vi "Info.vi"(8 "error in":errorcluster, 11 "Driver path":path) -> (0 "error out":errorcluster, 3 "Info":string)   [LabVIEW 2020, in "r307-python-labview-driver.lvlib"]
uses:
  r307-python-labview-driver.lvlib
panel:
  out "command line":string="cmc /c python \"%s\" ENROLL"
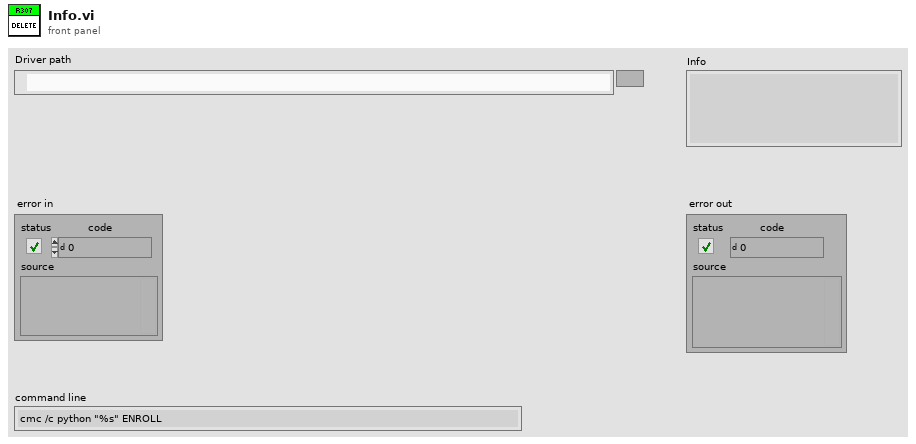
[diagram p1: front panel]
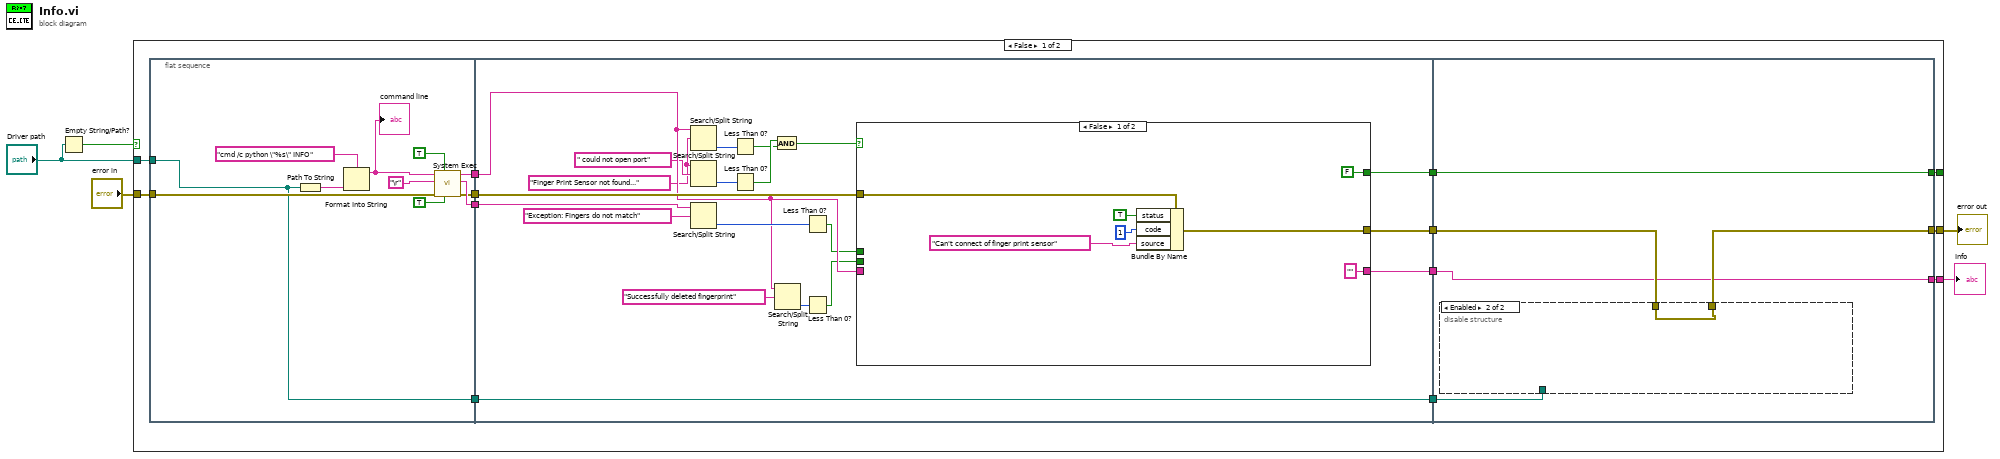
[diagram p0: block diagram]
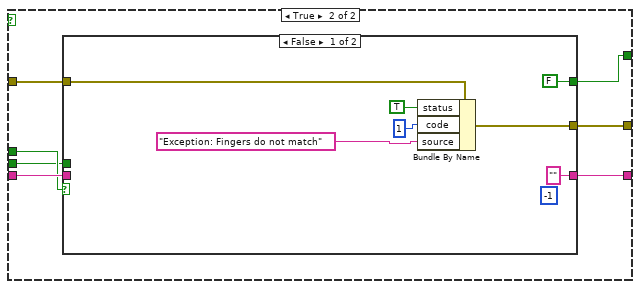
[diagram p2: hidden frame]
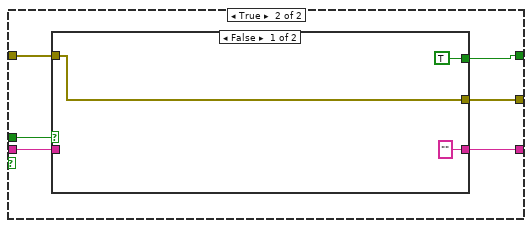
[diagram p3: hidden frame]
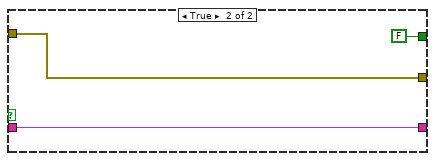
[diagram p4: hidden frame]
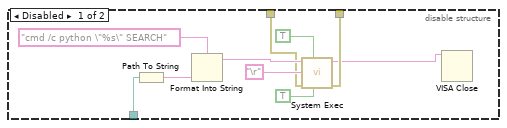
[diagram p5: hidden frame]
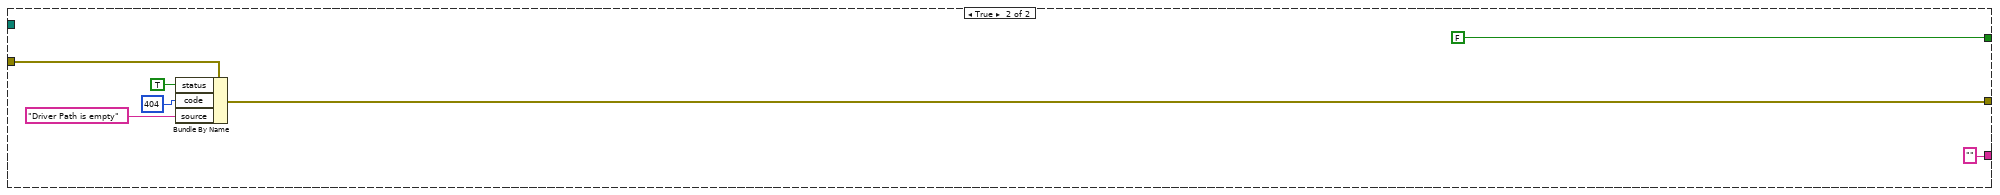
[diagram p6: hidden frame]
diagram:
  n1 = Empty String/Path?(string/path="Driver path") -> (empty?=w3:bool)
  n2 = case shown="False" w3 {
    tunnel: "Driver path" -> [w15 _]
    tunnel: "error in" -> [w14 w105]
    tunnel: [w13 w101] -> w4
    tunnel: [w12 FALSE ("Found")] -> _
    tunnel: [w7 "" ("standard output")] -> w1
    frame False {
      n3 = flat-sequence {
        tunnel: w15 -> [w19]
        tunnel: w14 -> [w21]
        tunnel: [w24] -> w18
        tunnel: [w20] -> w17
        tunnel: [w23] -> w16
        tunnel: [w19] -> w8
        tunnel: w18 -> [w48]
        tunnel: w17 -> [w47]
        tunnel: w16 -> [w41]
        tunnel: [w43] -> w11
        tunnel: [w39] -> w10
        tunnel: [w32] -> w9
        tunnel: w8 -> [w32]
        tunnel: [w30] -> w6
        tunnel: [w87] -> w12
        tunnel: [w84] -> w13
        tunnel: w11 -> [w85]
        tunnel: w10 -> [w87]
        tunnel: w9 -> [w86]
        tunnel: [w83] -> w7
        tunnel: w6 -> [w83]
        frame #0 {
          n4 = Path To String(path=w19) -> (string=w26:string)
          n5 = Format Into String(format string="cmd /c python \"%s\" INFO" ("command line"), w26) -> (resulting string=w27:string)  [unwired: 2 in, 1 out]
          "command line" <- w27
          n6 = call <vilib>:"System Exec.vi"("run minimized? (F)"=TRUE, "wait until completion? (T)"=TRUE, "error in (no error)"=w21, "standard input"="\r", "command line"=w27) -> ("error out"=w20:errorcluster, "standard error"=w24:string, "standard output"=w23:string)  [unwired: 3 in, 1 out]
        }
        frame #1 {
          w33 = "Finger Print Sensor not found..." ("search string/char (-)")
          n7 = Search/Split String(string=w41, search string/char (-)=w33) -> (offset of match=w46:i32)  [unwired: 1 in, 2 out]
          n8 = Search/Split String(string=w33, search string/char (-)=" could not open port") -> (offset of match=w38:i32)  [unwired: 1 in, 2 out]
          n9 = Search/Split String(string=w48, search string/char (-)="Exception: Fingers do not match") -> (offset of match=w49:i32)  [unwired: 1 in, 2 out]
          n10 = Less Than 0?(x=w46) -> (x < 0?=w36:bool)
          n11 = Less Than 0?(x=w38) -> (x < 0?=w37:bool)
          n12 = And(x=w37, y=w36) -> (x .and. y?=w35:bool)
          n13 = Search/Split String(string=w41, search string/char (-)="Successfully deleted fingerprint" ("string")) -> (offset of match=w45:i32)  [unwired: 1 in, 2 out]
          n14 = Less Than 0?(x=w49) -> (x < 0?=w40:bool)
          n15 = Less Than 0?(x=w45) -> (x < 0?=w31:bool)
          n16 = case shown="False" w35 {
            tunnel: w47 -> [w53 w63]
            tunnel: w41 -> [_ w61]
            tunnel: [w52 w62] -> w43
            tunnel: w40 -> [_ w60]
            tunnel: w31 -> [_ w59]
            tunnel: [FALSE ("Found") w58] -> w39
            tunnel: ["" ("standard output") w57] -> w30
            frame False {
              n17 = Bundle By Name(cluster=w53, "status"=TRUE, "code"=1, "source"="Can't connect of finger print sensor" ("search string/char (-)")) -> (w52:errorcluster)
            }
            frame True {
              n18 = case shown="False" w60 {
                tunnel: w63 -> [w70 w74]
                tunnel: [w67 w73] -> w62
                tunnel: w61 -> [_ w76]
                tunnel: w59 -> [_ w75]
                tunnel: [FALSE ("Found") w72] -> w58
                tunnel: ["" ("standard output") w71] -> w57
                frame False {
                  (unwired) -1 ("Enrolled ID")
                  n19 = Bundle By Name(cluster=w70, "status"=TRUE, "code"=1, "source"="Exception: Fingers do not match" ("search string/char (-)")) -> (w67:errorcluster)
                }
                frame True {
                  n20 = case shown="False" w75 {
                    tunnel: w76 -> [_ w80]
                    tunnel: w74 -> [w79 w82]
                    tunnel: [w79 w82] -> w73
                    tunnel: [TRUE ("Found") FALSE ("Found")] -> w72
                    tunnel: ["" ("standard output") w80] -> w71
                    frame False {
                    }
                    frame True {
                    }
                  }
                }
              }
            }
          }
        }
        frame #2 {
          n21 = disable-structure shown="Enabled" {
            disable-tunnel: w86 -> [w91 _]
            disable-tunnel: w85 -> [w90 w98]
            disable-tunnel: [w89 w98] -> w84
            frame Disabled {
              n22 = Path To String(path=w91) -> (string=w96:string)
              n23 = Format Into String(format string="cmd /c python \"%s\" SEARCH" ("command line"), w96) -> (resulting string=w97:string)  [unwired: 2 in, 1 out]
              n24 = call <vilib>:"System Exec.vi"("run minimized? (F)"=TRUE, "wait until completion? (T)"=TRUE, "error in (no error)"=w90, "standard input"="\r", "command line"=w97) -> ("error out"=w89:errorcluster, "standard output"=w88:string)  [unwired: 3 in, 2 out]
              n25 = VISA Close(VISA resource name=w88) -> ()  [unwired: 1 in, 1 out]
            }
            frame Enabled {
            }
          }
        }
      }
    }
    frame True {
      n26 = Bundle By Name(cluster=w105, "status"=TRUE, "code"=404, "source"="Driver Path is empty") -> (w101:errorcluster)
    }
  }
  "error out" <- w4
  "Info" <- w1
